vi "Panel.vi"(8 "error in (no error)":errorcluster, 10 "VI Panel Path":path, 11 "Panel in":refnum<class "Panel.lvclass">) -> (0 "error out":errorcluster, 3 "Panel out":refnum<class "Panel.lvclass">)   [LabVIEW 2018, in "Panel.lvclass"]
uses:
  Panel.lvclass
  Panel.lvclass/Panel.ctl
  setVIName.vi
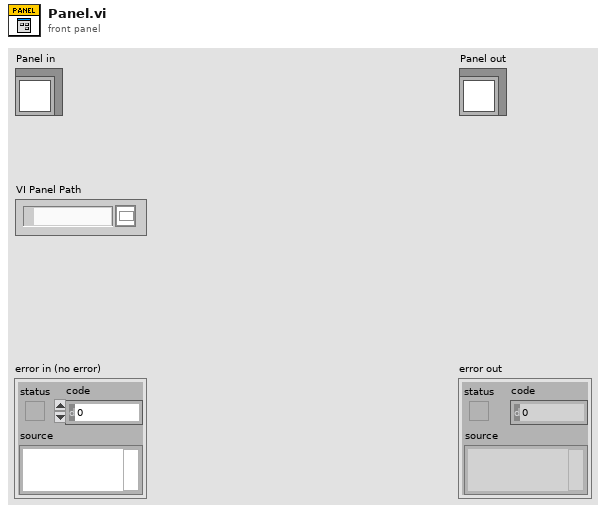
[diagram p1: front panel]
types:
  T1 = enum16{"Open Reference", "Launch VI", "Get VI Outputs"}
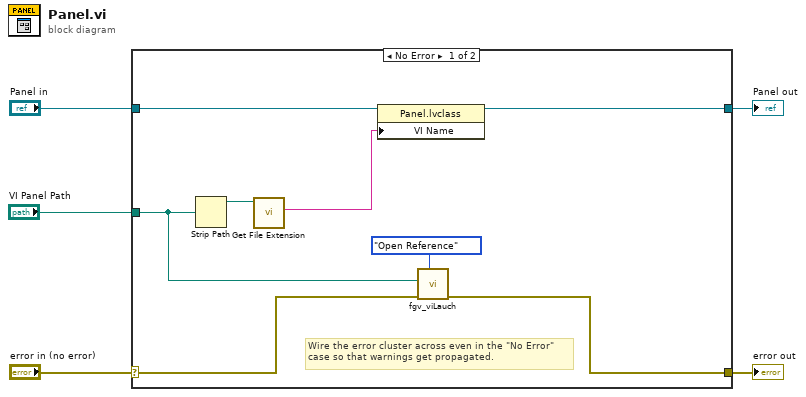
[diagram p0: block diagram]
diagram:
  n1 = case shown="No Error" "error in (no error)" {
    selector: "error in (no error)" -> [w9 w15]
    tunnel: [w8 w15] -> w4
    tunnel: [w12 w14] -> w2
    tunnel: "Panel in" -> [w13 w14]
    tunnel: "VI Panel Path" -> [w7 _]
    frame No Error {
      # "Wire the error cluster across even in the \"No Error\"\ncase so that warnings get propagated."
      n2 = Strip Path(path=w7) -> (stripped path=w11:path)  [unwired: 1 out]
      n3 = call <vilib>:"Get File Extension.vi"("file"=w11) -> ("lowercase file extension"=w10:string)  [unwired: 6 in, 4 out]
      n4 = property class="Panel.lvclass"(reference=w13, "VI Name"=w10) -> (reference out=w12:refnum<class "Panel.lvclass">)  [unwired: 1 in, 1 out]
      n5 = call "fgv_viLauch.vi"("Option"=T1."Open Reference", "Error In"=w9, "vi path"=w7) -> ("Error Out"=w8:errorcluster)  [unwired: 6 in, 2 out]
    }
    frame Error {
    }
  }
  "error out" <- w4
  "Panel out" <- w2
